vi "AIT 1553 - Build RT Message Properties.vi"(8 "error in (no error)":errorcluster, 10 "RT_Message":T1) -> (0 "error out":errorcluster, 1 "Tx-Rx  (T=Tx)":bool, 2 "name":string, 4 "Prop Names":string[](array[string]), 6 "Prop Values":variant[](array[variant]))   [LabVIEW 2013, in "AIT 1553 Custom Device.lvlib"]
uses:
  AIT 1553 Custom Device.lvlib
  Controls/1553_RT_Message.ctl
  Controls/1553 Param.ctl
  Controls and Global/Global.vi
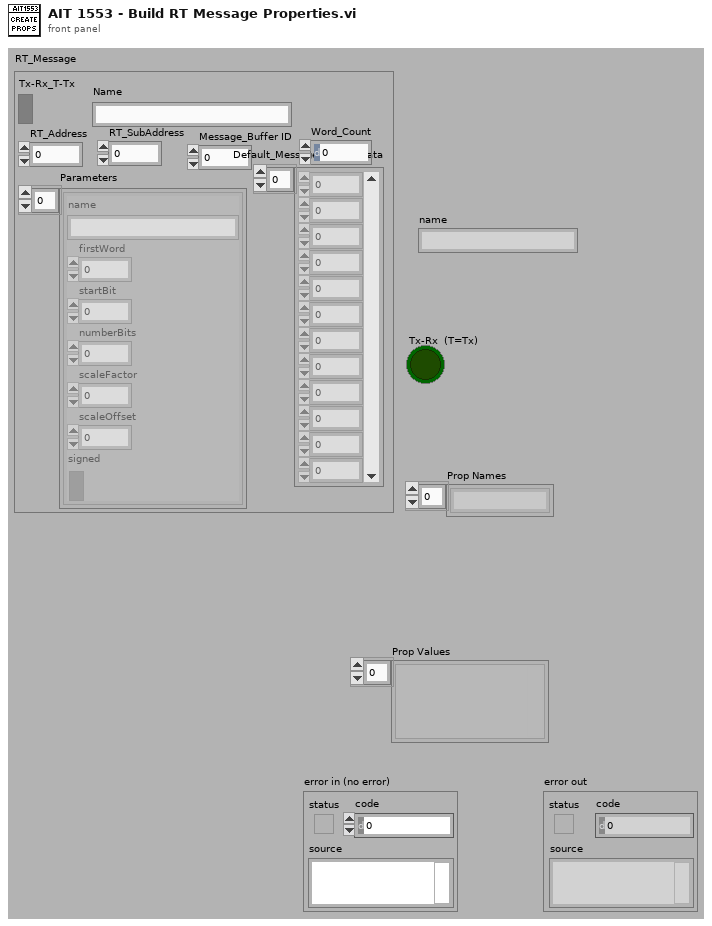
[diagram p1: front panel]
types:
  T1 = typedef "AIT 1553 Custom Device.lvlib/1553_RT_Message.ctl" = cluster{"RT_Address":u8, "RT_SubAddress":u8, "Tx-Rx_T-Tx":bool, "Parameters":T2[], "Message_Buffer ID":u16, "Default_Message_Buffer_Data":u16[], "Word_Count":u8, "Name":string}
  T2 = typedef "AIT 1553 Custom Device.lvlib/1553 Param.ctl" = cluster{"name":string, "firstWord":i32, "startBit":i32, "numberBits":i32, "scaleFactor":dbl, "scaleOffset":dbl, "signed":bool}
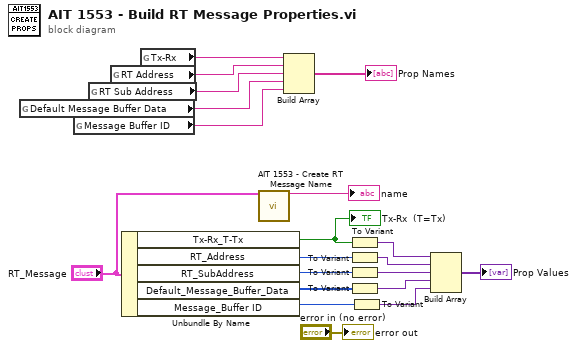
[diagram p0: block diagram]
diagram:
  n1 = global read "Global.vi" "Default Message Buffer Data"() -> (w9:string)
  n2 = global read "Global.vi" "Message Buffer ID"() -> (w6:string)
  n3 = global read "Global.vi" "RT Sub Address"() -> (w18:string)
  n4 = global read "Global.vi" "RT Address"() -> (w5:string)
  n5 = Unbundle By Name("RT_Message") -> ("Tx-Rx_T-Tx"=w12:bool, "RT_Address"=w13:u8, "RT_SubAddress"=w14:u8, "Default_Message_Buffer_Data"=w8:u16[], "Message_Buffer ID"=w4:u16)
  "Tx-Rx  (T=Tx)" <- w12
  n6 = global read "Global.vi" "Tx-Rx"() -> (w20:string)
  n7 = call "AIT 1553 - Create RT Message Name.vi"("RT_Message"="RT_Message") -> ("Message Name"=→"name":string)  [unwired: 13 in, 1 out]
  n8 = Build Array(w20, w5, w18, w9, w6) -> (→"Prop Names":string[])
  n9 = To Variant(anything=w12) -> (Variant=w15:variant)
  n10 = To Variant(anything=w13) -> (Variant=w16:variant)
  n11 = To Variant(anything=w14) -> (Variant=w17:variant)
  n12 = To Variant(anything=w8) -> (Variant=w7:variant)
  n13 = To Variant(anything=w4) -> (Variant=w3:variant)
  n14 = Build Array(w15, w16, w17, w7, w3) -> (→"Prop Values":variant[])
  "error out" <- "error in (no error)"
